vi "SWERVE_TRAJECTORY_READFILE_BEGIN.vi"(11 "Trajectory File Name":string="test_path.wpilib.json") -> (0 "error out":errorcluster, 2 "Trajectory Items":i32, 3 "TotalTImeSecs":dbl)   [LabVIEW 2020]
uses:
  <vilib>/Rock Robotics/WPI/ThirdParty/JAS_Junk/TrajLib/Trajectory_Library.lvlib
panel:
  # "Relative or absolute trajectory\nfile name"
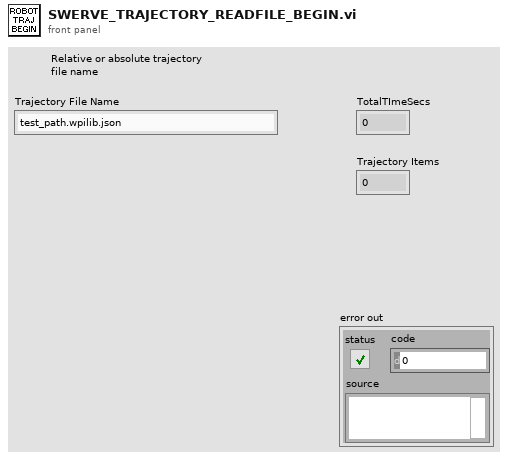
[diagram p1: front panel]
types:
  T1 = typedef "Trajectory_Library.lvlib/TRAJECTORY.ctl" = cluster{"TotalTImeSecs":dbl, "States":T2[]}
  T2 = typedef "Trajectory_Library.lvlib/TRAJ_STATE.ctl" = cluster{"TimeSeconds":dbl, "Velocity":dbl, "Acceleration":dbl, "POSE":T3, "Curvature":dbl}
  T3 = typedef "Trajectory_Library.lvlib/POSE2D.ctl" = cluster{"TRANSLATION":T4, "ROTATION":T5}
  T4 = typedef "Trajectory_Library.lvlib/TRANSLATION2D.ctl" = cluster{"X":dbl, "Y":dbl}
  T5 = typedef "Trajectory_Library.lvlib/ROTATION2D.ctl" = cluster{"VALUE":dbl, "COS":dbl, "SIN":dbl}
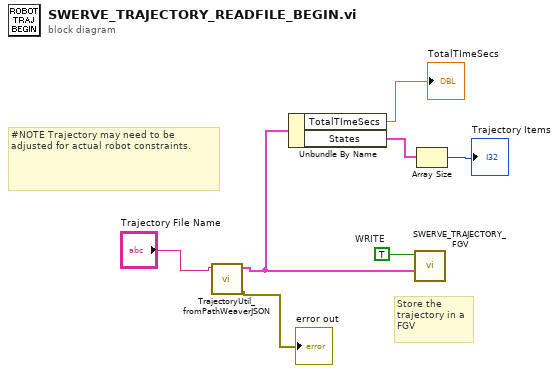
[diagram p0: block diagram]
diagram:
  w7 = TRUE  # WRITE
  # "#NOTE Trajectory may need to be adjusted for actual robot constraints."
  # "Store the\ntrajectory in a \nFGV"
  n1 = call <vilib>:"TrajectoryUtil_fromPathWeaverJSON.vi"("FileName"="Trajectory File Name") -> ("error out"=→"error out":errorcluster, "outTRAJECTORY"=w1:T1)  [unwired: 8 in, 1 out]
  n2 = Unbundle By Name(w1) -> ("TotalTImeSecs"=→"TotalTImeSecs":dbl, "States"=w5:T2[])
  n3 = call "SWERVE_TRAJECTORY_FGV.vi"("inTRAJECTORY"=w1, "WRITE"=w7) -> ()  [unwired: 9 in, 1 out]
  n4 = Array Size(array=w5) -> (size(s)=→"Trajectory Items":i32)
